vi "sendarray.vi"(6 "addr/port":cluster{"address":string, "port":i32}={"address"="127.0.0.1", "port"=31415}, 8 "error in (no error)":errorcluster, 10 "numerical array":dbl[](array[numeric]), 11 "command string":string) -> (0 "error out":errorcluster, 2 "bytes written":i32, 3 "connection ID out":refnum<k5>)   [LabVIEW 2015]
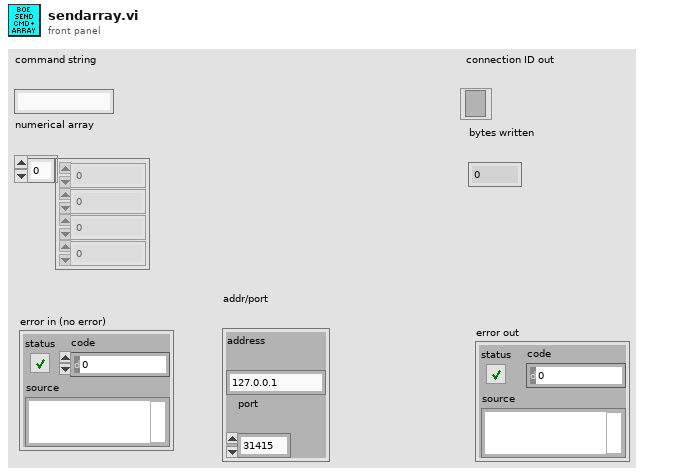
[diagram p1: front panel]
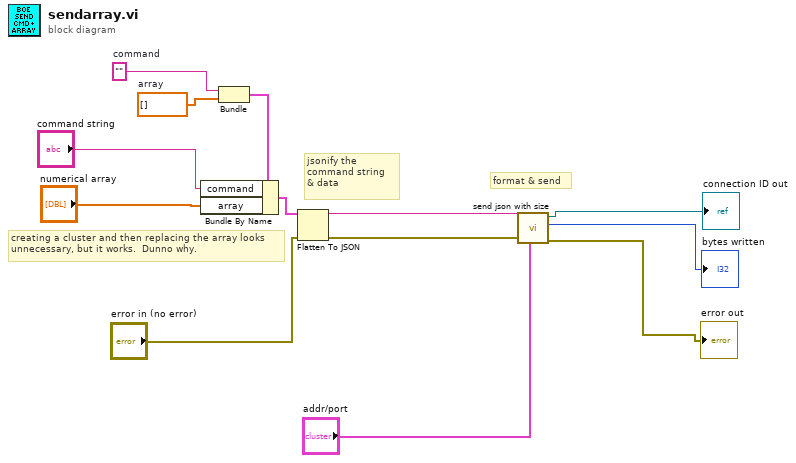
[diagram p0: block diagram]
diagram:
  w12 = ""  # command
  w13 = dbl[] []  # array
  # "format & send"
  # "creating a cluster and then replacing the array looks\nunnecessary, but it works.  Dunno why."
  # "jsonify the \ncommand string \n& data"
  n1 = Bundle("command"=w12, "array"=w13) -> (w11:cluster{"command":string, "array":dbl[]})  [unwired: 1 in]
  n2 = Bundle By Name(cluster=w11, "command"="command string", "array"="numerical array") -> (w8:cluster{"command":string, "array":dbl[]})
  n3 = Flatten To JSON(anything=w8, error in (no error)="error in (no error)") -> (JSON string=w6:string, 11:w5:errorcluster)  [unwired: 1 in]
  n4 = call "send json with size.vi"("addr/port"="addr/port", "error in"=w5, "json string"=w6) -> ("error out"=→"error out":errorcluster, "bytes written"=→"bytes written":i32, "connection ID out"=→"connection ID out":refnum<k5>)  [unwired: 6 in]
